vi "Table, Set Text Plain.vi"(6 "error in":errorcluster, 9 "Tbl Refnum":refnum<vi>) -> (0 "error out":errorcluster, 3 "Tbl Refnum out":refnum<vi>)   [LabVIEW 2010]
doc: "This function sets the active table cell font attribute to bold."
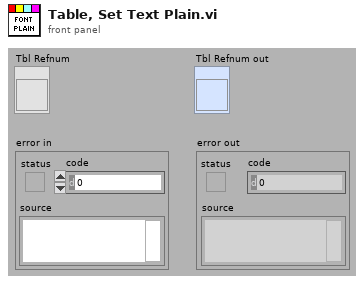
[diagram p1: front panel]
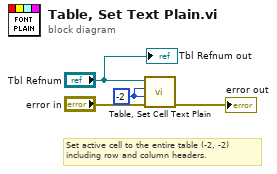
[diagram p0: block diagram]
diagram:
  w1 = -2 ("row (0)")
  # "Set active cell to the entire table (-2, -2)\nincluding row and column headers."
  n1 = call "Table, Set Cell Text Plain.vi"("error in"="error in", "col (0)"=w1, "row (0)"=w1, "Tbl Refnum"="Tbl Refnum") -> ("error out"=→"error out":errorcluster)  [unwired: 2 in, 3 out]
  "Tbl Refnum out" <- "Tbl Refnum"
